vi "AttrGetState.vi"(8 "error in":errorcluster, 11 "CanHandleIn":T1) -> (0 "error out":errorcluster, 2 "State":T2, 3 "CanHandleOut":T1)   [LabVIEW 2011, in "Konvolucio MCAN120803.lvlib"]
doc: "Get adapter current state.\nDefault state is SDEV_IDLE."
uses:
  <instrlib>/Konvolucio MCAN120803/Konvolucio MCAN120803.lvlib
  <instrlib>/Konvolucio MCAN120803/Types/StateType.ctl
  <instrlib>/Konvolucio MCAN120803/Types/CanHandleType.ctl
  C:/Program Files/National Instruments/LabVIEW 2011/instr.lib/Konvolucio MCAN120803/Private/Konvolucio.MCAN120803.API.dll
  Private/Konvolucio.MCAN120803.API.dll
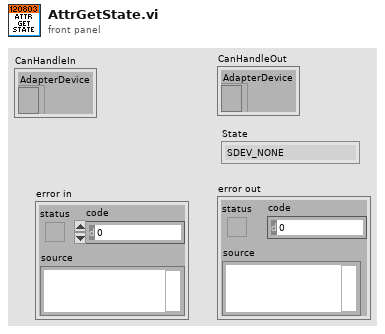
[diagram p1: front panel]
types:
  T1 = typedef "Konvolucio MCAN120803.lvlib/CanHandleType.ctl" = cluster{"AdapterDevice":refnum<k24>}
  T2 = typedef "Konvolucio MCAN120803.lvlib/StateType.ctl" = enum16{"SDEV_NONE", "SDEV_START", "SDEV_STOP", "SDEV_RESET", "SDEV_FAIL", "SDEV_IDLE"}
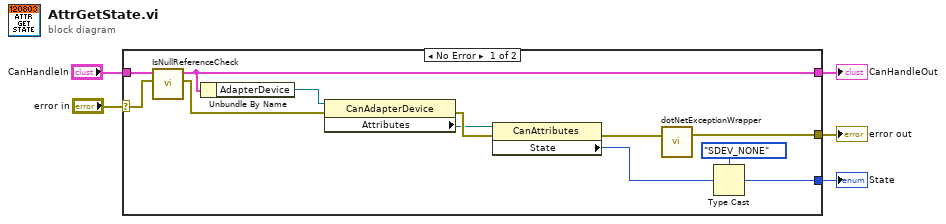
[diagram p0: block diagram]
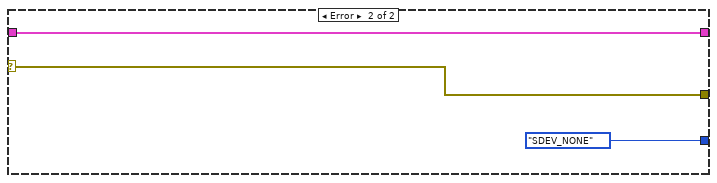
[diagram p2: hidden frame]
diagram:
  n1 = case shown="No Error" "error in" {
    selector: "error in" -> [w10 w20]
    tunnel: [w14 w20] -> w5
    tunnel: [w16 StateType."SDEV_NONE" ("MCanState")] -> w3
    tunnel: "CanHandleIn" -> [w11 w18]
    tunnel: [w12 w18] -> w1
    frame No Error {
      n2 = call <instrlib>:"IsNullReferenceCheck.vi"("error in"=w10, "MCanHandleIn"=w11) -> ("error out"=w8:errorcluster, "MCanHandleOut"=w12:T1)  [unwired: 5 in]
      n3 = Unbundle By Name(w12) -> ("AdapterDevice"=w9:refnum<k24>)
      n4 = property class="CanAdapterDevice"(reference=w9, error in=w8) -> (error out=w7:errorcluster, "Attributes"=w6:refnum<k24>)  [unwired: 1 out]
      n5 = property class="CanAttributes"(reference=w6, error in=w7) -> (error out=w13:errorcluster, "State"=w15:u32)  [unwired: 1 out]
      n6 = call <instrlib>:"dotNetExceptionWrapper.vi"("error in"=w13) -> ("error out"=w14:errorcluster)  [unwired: 2 in]
      n7 = Type Cast(type=StateType."SDEV_NONE" ("MCanState"), x=w15) -> (*(type *) &x=w16:T2)
    }
    frame Error {
    }
  }
  "error out" <- w5
  "State" <- w3
  "CanHandleOut" <- w1
